vi "TearDown.vi"(0 "Application Ref":refnum<vi>, 5 "VI in":refnum<vi>, 11 "error in (no error)":errorcluster) -> (15 "error out":errorcluster)   [LabVIEW 2016, in "DronaTest.lvlib"]
uses:
  DronaTest.lvlib
  APIs/Stimulus/VI/CloseVI.vi
  APIs/Assert/AssertVI/Execution/AssertVIExecIdle.vi
  Drona.lvlib
  APIs/Stimulus/VI/VI.lvlib
  APIs/Assert/AssertVI/AssertVI.lvlib
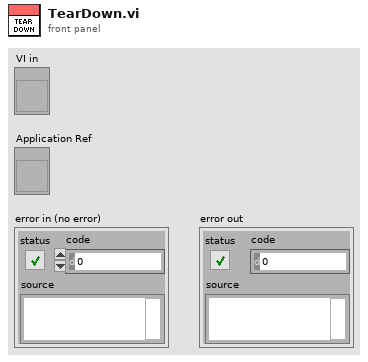
[diagram p1: front panel]
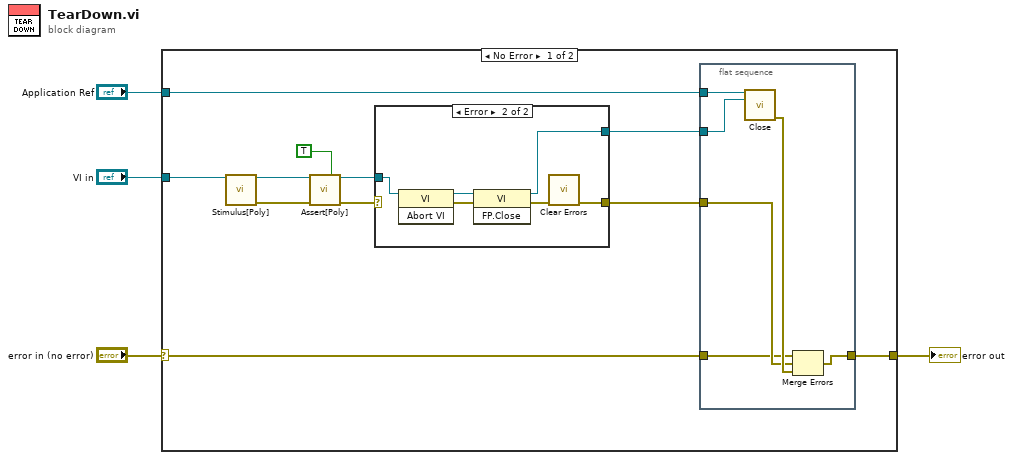
[diagram p0: block diagram]
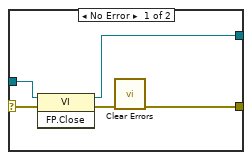
[diagram p2: hidden frame]
diagram:
  n1 = case shown="No Error" "error in (no error)" {
    selector: "error in (no error)" -> [w5 w33]
    tunnel: "VI in" -> [w15 _]
    tunnel: [w14 w33] -> w3
    tunnel: "Application Ref" -> [w13 _]
    frame No Error {
      n2 = call-poly "Stimulus[Poly].vi"("VI Reference In"=w15) -> ("VI Reference Out"=w11:refnum<vi>, "error out"=w12:errorcluster)  [unwired: 13 in]
      n3 = call-poly "Assert[Poly].vi"("VI Reference In"=w11, "Assert Only? (F)"=TRUE, "Error In"=w12) -> ("VI Reference Out"=w6:refnum<vi>, "Error Out"=w8:errorcluster)  [unwired: 10 in, 1 out]
      n4 = case shown="Error" w8 {
        selector: w8 -> [w20 _]
        tunnel: [w16 w24] -> w9
        tunnel: [w17 w25] -> w7
        tunnel: w6 -> [w18 w22]
        frame No Error {
          n5 = invoke class="VI" method="FP.Close"(reference=w18, error in=w20) -> (reference out=w17:refnum<vi>, error out=w19:errorcluster)  [unwired: 1 in, 1 out]
          n6 = call <vilib>:"Clear Errors.vi"("error in (no error)"=w19) -> ("error out"=w16:errorcluster)  [unwired: 5 in, 1 out]
        }
        frame Error {
          n7 = invoke class="VI" method="Abort VI"(reference=w22) -> (reference out=w21:refnum<vi>, error out=w23:errorcluster)  [unwired: 2 in, 1 out]
          n8 = invoke class="VI" method="FP.Close"(reference=w21, error in=w23) -> (reference out=w25:refnum<vi>, error out=w26:errorcluster)  [unwired: 1 in, 1 out]
          n9 = call <vilib>:"Clear Errors.vi"("error in (no error)"=w26) -> ("error out"=w24:errorcluster)  [unwired: 5 in, 1 out]
        }
      }
      n10 = flat-sequence {
        tunnel: [w29] -> w14
        tunnel: w13 -> [w31]
        tunnel: w7 -> [w30]
        tunnel: w9 -> [w28]
        tunnel: w5 -> [w27]
        frame #0 {
          n11 = call "Close.vi"("Application Ref"=w31, "VI Reference"=w30) -> ("error out"=w32:errorcluster)  [unwired: 13 in]
          n12 = Merge Errors(w27, w28, w32) -> (w29:errorcluster)
        }
      }
    }
    frame Error {
    }
  }
  "error out" <- w3
